vi "Music.vi"(11 "path":path) -> (3 "data":waveform(dbl)[](array[waveform]))   [LabVIEW 2017]
panel:
  out "error out":errorcluster
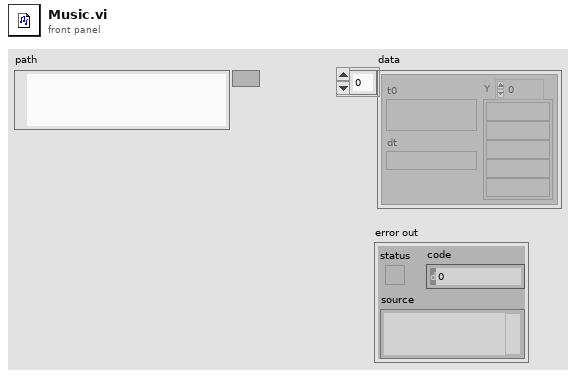
[diagram p1: front panel]
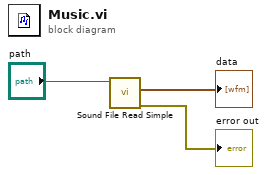
[diagram p0: block diagram]
diagram:
  n1 = call <vilib>:"Sound File Read Simple.vi"("path"="path") -> ("error out"=→"error out":errorcluster, "data"=→"data":waveform(dbl)[])  [unwired: 7 in, 2 out]
